vi "MecaDrivePoseEst2_InterpRecord_Interp.vi"(6 "Extra":variant, 9 "Time Fraction":dbl, 10 "End Input 2":variant, 11 "Input 1":variant) -> (3 "Interp Output":variant)   [LabVIEW 2019, in "Trajectory_Library.lvlib"]
doc: "Performs interpolation for a SwerveDrivePoseEstimator2 Interpolation Record.\n\nThis is an internal routine. It should NOT be used by end users."
uses:
  Trajectory_Library.lvlib
  <vilib>/Analysis/Matrix/Datatypes/RealMatrix.ctl
  <vilib>/Analysis/Matrix/NI_Matrix.lvlib
  TypeDef/TRANSLATION2D.ctl
  TypeDef/MECA_DRIVE_KINEMATICS.ctl
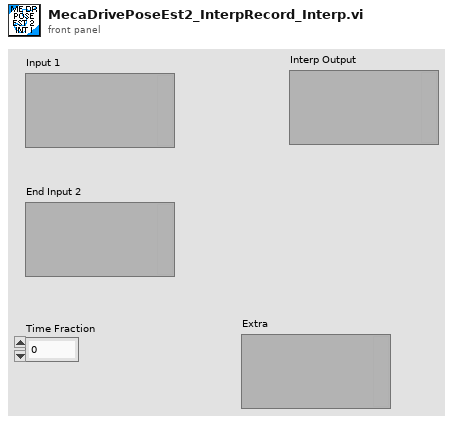
[diagram p1: front panel]
types:
  T1 = typedef "Trajectory_Library.lvlib/MECA_DRIVE_POSE_EST2_INTERP_RECORD.ctl" = cluster{"PoseMeters":T2, "GyroAngle":T4, "ModulePositions":T5}
  T2 = typedef "Trajectory_Library.lvlib/POSE2D.ctl" = cluster{"TRANSLATION":T3, "ROTATION":T4}
  T3 = typedef "Trajectory_Library.lvlib/TRANSLATION2D.ctl" = cluster{"X":dbl, "Y":dbl}
  T4 = typedef "Trajectory_Library.lvlib/ROTATION2D.ctl" = cluster{"VALUE":dbl, "COS":dbl, "SIN":dbl}
  T5 = typedef "Trajectory_Library.lvlib/MECA_WHEEL_POSITIONS.ctl" = cluster{"FrontLeft":dbl, "FrontRight":dbl, "RearLeft":dbl, "RearRight":dbl, "P":bool}
  T6 = typedef "Trajectory_Library.lvlib/MECA_DRIVE_KINEMATICS.ctl" = cluster{"FrontLeft":T3, "FrontRight":T3, "RearLeft":T3, "RearRight":T3, "InverseKinematics":T7, "ForwardKinematics":T7, "PrevCoR":T3}
  T7 = typedef "NI_Matrix.lvlib/RealMatrix.ctl" = dbl[][]
  T8 = typedef "Trajectory_Library.lvlib/TWIST2D.ctl" = cluster{"dX":dbl, "dY":dbl, "dTHETA":dbl}
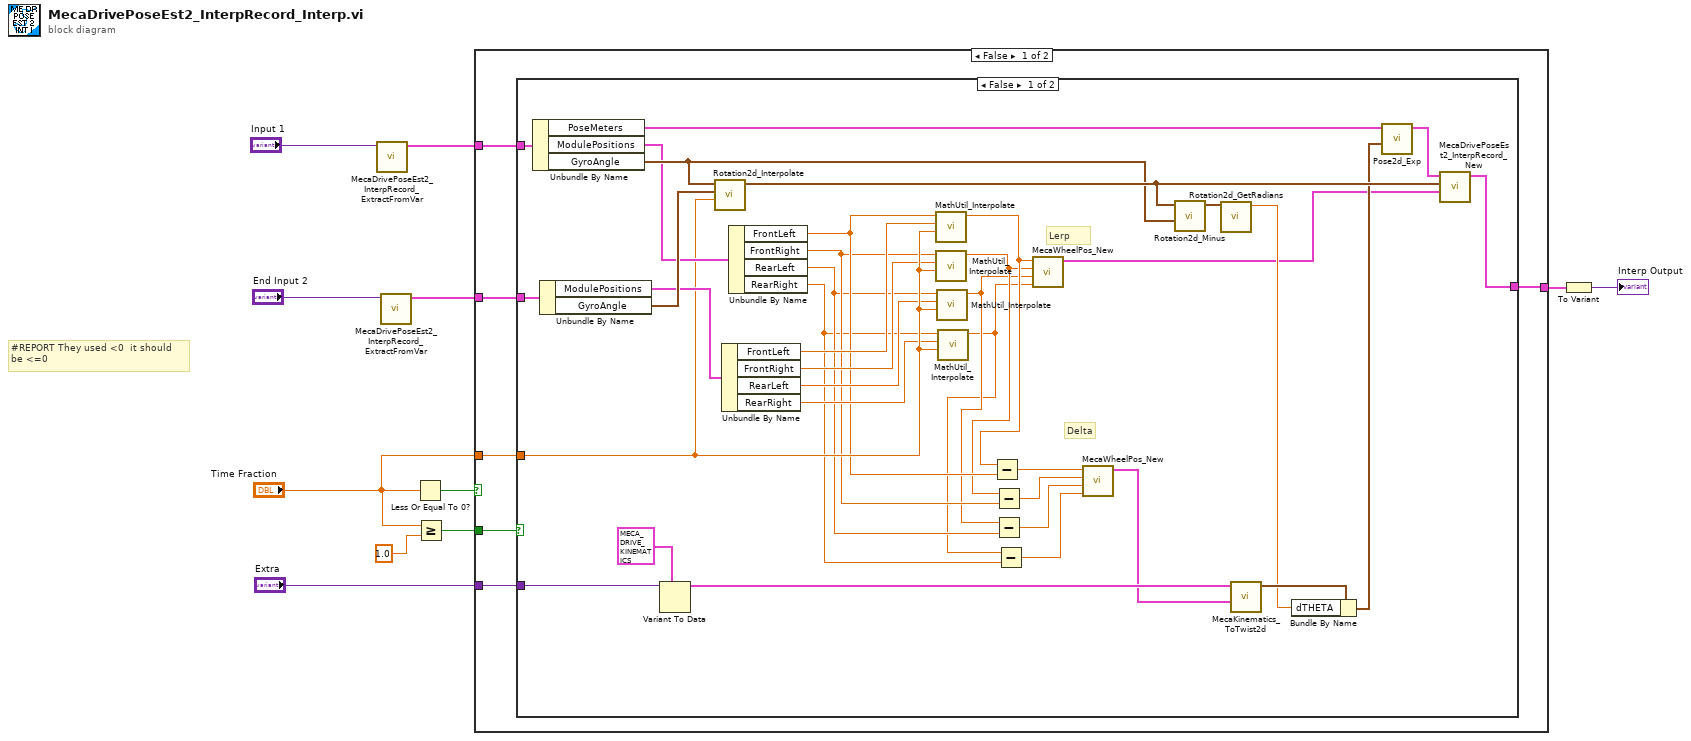
[diagram p0: block diagram]
diagram:
  # "#REPORT They used <0  it should\nbe <=0"
  n1 = call "MecaDrivePoseEst2_InterpRecord_ExtractFromVar.vi"("OutputVariant"="Input 1") -> ("out InterpRecord"=w3:T1)  [unwired: 9 in, 1 out]
  n2 = call "MecaDrivePoseEst2_InterpRecord_ExtractFromVar.vi"("OutputVariant"="End Input 2") -> ("out InterpRecord"=w1:T1)  [unwired: 9 in, 1 out]
  n3 = Less Or Equal To 0?(x="Time Fraction") -> (x <= 0?=w11:bool)
  n4 = Greater Or Equal?(x="Time Fraction", y=1.0) -> (x >= y?=w7:bool)
  n5 = case shown="False" w11 {
    tunnel: [w16 w55] -> w9
    tunnel: w3 -> [w14 w55]
    tunnel: w7 -> [w17 _]
    tunnel: w1 -> [w15 _]
    tunnel: "Time Fraction" -> [w13 _]
    tunnel: "Extra" -> [w12 _]
    frame False {
      n6 = case shown="False" w17 {
        tunnel: [w39 w54] -> w16
        tunnel: w15 -> [w52 w54]
        tunnel: w14 -> [w53 _]
        tunnel: w13 -> [w32 _]
        tunnel: w12 -> [w50 _]
        frame False {
          # "Delta"
          # "Lerp"
          n7 = Unbundle By Name(w53) -> ("PoseMeters"=w42:T2, "ModulePositions"=w38:T5, "GyroAngle"=w45:T4)
          n8 = Unbundle By Name(w52) -> ("ModulePositions"=w37:T5, "GyroAngle"=w51:T4)
          n9 = Variant To Data(type=T6 {"FrontLeft"={"X"=0.0, "Y"=0.0}, "FrontRight"={"X"=0.0, "Y"=0.0}, "RearLeft"={"X"=0.0, "Y"=0.0}, "RearRight"={"X"=0.0, "Y"=0.0}, "InverseKinematics"=[[0.0, 1.0, -1.0, 0.0], [0.0, 1.0, 1.0, 0.0], [0.0, 1.0, 1.0, 0.0], [0.0, 1.0, -1.0, 0.0]], "ForwardKinematics"=[[0.0, 1.0, -1.0, 0.0], [0.0, 1.0, 1.0, 0.0], [0.0, 1.0, 1.0, 0.0], [0.0, 1.0, -1.0, 0.0]], "PrevCoR"={"X"=0.0, "Y"=0.0}} ("MECA_DRIVE_KINEMATICS"), Variant=w50) -> (data=w48:T6)  [unwired: 1 in, 1 out]
          n10 = call "Rotation2d_Interpolate.vi"("T"=w32, "EncValue ROTATION"=w51, "in ROTATION"=w45) -> ("Interpolated ROTATION"=w46:T4)  [unwired: 8 in]
          n11 = Unbundle By Name(w37) -> ("FrontLeft"=w35:dbl, "FrontRight"=w31:dbl, "RearLeft"=w30:dbl, "RearRight"=w29:dbl)
          n12 = Unbundle By Name(w38) -> ("FrontLeft"=w28:dbl, "FrontRight"=w27:dbl, "RearLeft"=w26:dbl, "RearRight"=w25:dbl)
          n13 = call "MathUtil_Interpolate.vi"("T"=w32, "EndValue"=w35, "StartValue"=w28) -> ("InterpolatedValue"=w21:dbl)  [unwired: 8 in]
          n14 = call "MathUtil_Interpolate.vi"("T"=w32, "EndValue"=w31, "StartValue"=w27) -> ("InterpolatedValue"=w20:dbl)  [unwired: 8 in]
          n15 = call "MathUtil_Interpolate.vi"("T"=w32, "EndValue"=w30, "StartValue"=w26) -> ("InterpolatedValue"=w19:dbl)  [unwired: 8 in]
          n16 = call "MathUtil_Interpolate.vi"("T"=w32, "EndValue"=w29, "StartValue"=w25) -> ("InterpolatedValue"=w18:dbl)  [unwired: 8 in]
          n17 = Subtract(x=w21, y=w28) -> (x-y=w33:dbl)
          n18 = Subtract(x=w20, y=w27) -> (x-y=w24:dbl)
          n19 = Subtract(x=w19, y=w26) -> (x-y=w23:dbl)
          n20 = Subtract(x=w18, y=w25) -> (x-y=w22:dbl)
          n21 = call "MecaWheelPos_New.vi"("RearRightPosition"=w18, "RearLeftPosition"=w19, "FrontRightPosition"=w20, "FrontLeftPosition"=w21) -> ("MECA_WHEEL_POSITIONS"=w36:T5)  [unwired: 7 in]
          n22 = call "MecaWheelPos_New.vi"("RearRightPosition"=w22, "RearLeftPosition"=w23, "FrontRightPosition"=w24, "FrontLeftPosition"=w33) -> ("MECA_WHEEL_POSITIONS"=w34:T5)  [unwired: 7 in]
          n23 = call "Rotation2d_Minus.vi"("other ROTATION"=w45, "in ROTATION"=w46) -> ("out ROTATION"=w44:T4)  [unwired: 9 in]
          n24 = call "Rotation2d_GetRadians.vi"("in ROTATION"=w44) -> ("AngleRadians"=w43:dbl)  [unwired: 10 in]
          n25 = call "MecaKinematics_ToTwist2d.vi"("Wheel Deltat Positions"=w34, "in MECA_DRIVE_KINEMATICS"=w48) -> ("Twist2d"=w47:T8)  [unwired: 9 in]
          n26 = Bundle By Name(cluster=w47, "dTHETA"=w43) -> (w40:T8)
          n27 = call "Pose2d_Exp.vi"("TWIST"=w40, "POSE"=w42) -> ("UpdatedPose"=w41:T2)  [unwired: 9 in]
          n28 = call "MecaDrivePoseEst2_InterpRecord_New.vi"("ModulePositions"=w36, "GyroAngle"=w46, "M_POSE_Meters"=w41) -> ("MECA_DRIVE_POSE_EST2_INTERP_RECORD"=w39:T1)  [unwired: 8 in]
        }
        frame True {
        }
      }
    }
    frame True {
    }
  }
  n29 = To Variant(anything=w9) -> (Variant=→"Interp Output":variant)
